vi "Constructor.vi"(5 "TimeZoneInfoId":string, 6 "MeasureExecutionStatus":T1=enum."NOT_COMPLETED", 7 "MeasureTime":timestamp, 8 "error in":errorcluster, 10 "Value":bool, 11 "Name":string) -> (0 "error out":errorcluster, 3 "BooleanMeasure":refnum<class "BooleanMeasure.lvclass">)   [LabVIEW 2021, in "ProligentXMLGenerator.lvlib" / "BooleanMeasure.lvclass"]
uses:
  BooleanMeasure.lvclass
  BooleanMeasure.lvclass/BooleanMeasure.ctl
  Measure/Measure.lvclass
  Base/MeasureKind/Value.ctl
  Base/MeasureKind/MeasureKind.lvclass
  Data.ctl
  Base/Boolean/Boolean.lvclass
  C:/Projects/proligent-xml-generator-labview/src/ProligentXMLGenerator/Measure/Measure/Measure.lvclass
  C:/Projects/proligent-xml-generator-labview/src/ProligentXMLGenerator/Measure/BooleanMeasure/BooleanMeasure.lvclass
  Base/ExecutionStatus/Value.ctl
  Base/ExecutionStatus/ExecutionStatus.lvclass
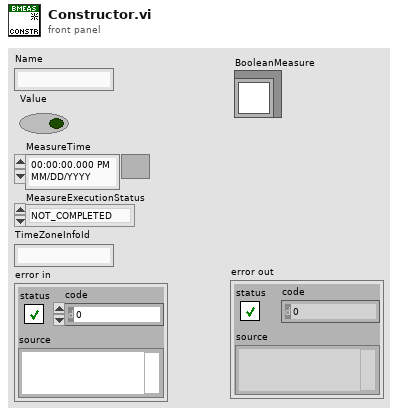
[diagram p1: front panel]
types:
  T1 = typedef "ProligentXMLGenerator.lvlib/ExecutionStatus.lvclass/Value.ctl" = enum16{"PASS", "FAIL", "NOT_COMPLETED", "ABORTED"}
  T2 = typedef "ProligentXMLGenerator.lvlib/BooleanMeasure.lvclass/Data.ctl" = cluster{"Value":refnum<class "Boolean.lvclass">}
  T3 = typedef "ProligentXMLGenerator.lvlib/MeasureKind.lvclass/Value.ctl" = enum16{"REAL", "BOOL", "INTEGER", "STRING", "DATETIME"}
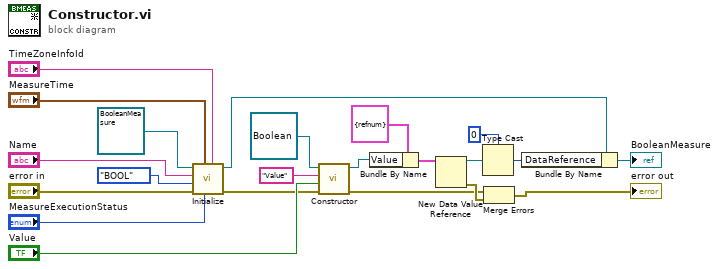
[diagram p0: block diagram]
diagram:
  n1 = call "Initialize.vi"("TimeZoneInfoId"="TimeZoneInfoId", "MeasureExecutionStatus"="MeasureExecutionStatus", "MeasureTime"="MeasureTime", "error in"="error in", "Type"=Value."BOOL", "Name"="Name", "Measure in"=refnum<class "BooleanMeasure.lvclass"> refnum ("ProligentResultProcessor:BooleanMeasure")) -> ("error out"=w7:errorcluster, "Measure out"=w17:refnum<class "BooleanMeasure.lvclass">)  [unwired: 3 in]
  n2 = call-dynamic "Constructor.vi"("error in"=w7, "Value"="Value", "Name"="Value", "Boolean in"=refnum<class "Boolean.lvclass"> refnum ("ProligentResultProcessor:Boolean")) -> ("error out"=w6:errorcluster, "Boolean out"=w3:refnum<class "Boolean.lvclass">)  [unwired: 6 in]
  n3 = Bundle By Name(cluster=T2 {"Value"=refnum} ("Data"), "Value"=w3) -> (w5:T2)
  n4 = New Data Value Reference(data value=w5) -> (data value reference=w18:refnum<data-value>, error out=w21:errorcluster)  [unwired: 1 in]
  n5 = Type Cast(type=u64 0, x=w18) -> (*(type *) &x=w20:u64)
  n6 = Merge Errors(w6, w21) -> (→"error out":errorcluster)
  n7 = Bundle By Name(cluster=w17, "DataReference"=w20) -> (→"BooleanMeasure":refnum<class "BooleanMeasure.lvclass">)
